vi "Select Session.vi"(10 "Input Session":refnum<class "Session.lvclass">, 11 "Output Session":refnum<class "Session.lvclass">) -> (2 "Session":refnum<class "Session.lvclass">)   [LabVIEW 2020, in "HTTP Server.lvlib" / "Server.lvclass"]
uses:
  Server.lvclass
  Server.lvclass/Server.ctl
  Session/Session.lvclass
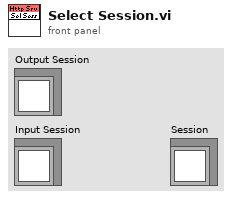
[diagram p1: front panel]
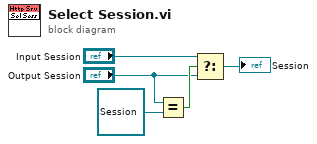
[diagram p0: block diagram]
diagram:
  n1 = Equal?(x="Output Session", y=refnum<class "Session.lvclass"> refnum) -> (x = y?=w4:bool)
  n2 = Select(t="Input Session", s=w4, f="Output Session") -> (s? t:f=→"Session":refnum<class "Session.lvclass">)
